vi "Time Delay (3).vi"(9 "Time Delay":u32=1000, 10 "Boolean in":bool) -> (2 "Boolean out":bool)   [LabVIEW 2016]
panel:
  out "FalseBtm Safety":u32
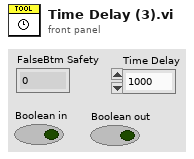
[diagram p1: front panel]
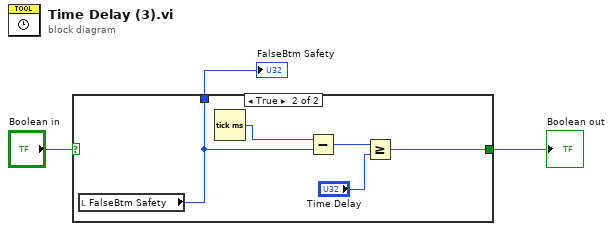
[diagram p0: block diagram]
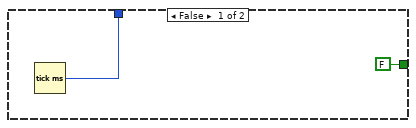
[diagram p2: hidden frame]
diagram:
  n1 = case shown="True" "Boolean in" {
    tunnel: [w5 w6] -> w2
    tunnel: [FALSE w8] -> w3
    frame False {
      n2 = Tick Count (ms)() -> (millisecond timer value=w5:u32)
    }
    frame True {
      n3 = local read "FalseBtm Safety"() -> (w6:u32)
      n4 = Tick Count (ms)() -> (millisecond timer value=w10:u32)
      n5 = Subtract(x=w10, y=w6) -> (x-y=w9:u32)
      n6 = Greater Or Equal?(x=w9, y="Time Delay") -> (x >= y?=w8:bool)
    }
  }
  "FalseBtm Safety" <- w2
  "Boolean out" <- w3
